vi "RoomJasonTest.vi"() -> (0 "error out":errorcluster, 2 "Pass":bool)   [LabVIEW 2015]
uses:
  Flags/ColorEnum.ctl
  NurseStation/TypeDef/SelectedRoom.ctl
  Flags/ColorFlags.ctl
  Room/Room.lvclass/Room.ctl
  Room/Write Beacon Id.vi
  Room/Write BedVacant.vi
  Room/Write InRoomPersonnel.vi
  Room/Write RoomRequests.vi
  Room/Read Beacon Id.vi
  Room/Read BedVacant.vi
  Room/Read InRoomPersonnel.vi
  Room/Read Room Number.vi
  Room/Read RoomRequests.vi
  Room/Read Flags.lvclass.vi
  Flags/Flags.lvclass
  Room/Room.lvclass
panel:
  out "String":string
  in  "RoomRequests":string[](array[string])=["Cleanning"]
  in  "InRoomPersonnel":string[](array[string])=["Dr Y"]
  in  "BedVacant":bool
  in  "Beacon Id":string="test"
  out "After Json":T1={"Room Number"=0, "RoomNumFlags"={"Flag State"=[1, 3, 5, 7]}, "BedVacant"=FALSE, "InRoomPersonnel"=[], "RoomRequests"=[]}
  out "Before Json":T1={"Room Number"=0, "RoomNumFlags"={"Flag State"=[1, 3, 5, 7]}, "BedVacant"=FALSE, "InRoomPersonnel"=[], "RoomRequests"=[]}
  in  "Color":T3[](array[typedef])=[enum."Red", enum."Blue", enum."Green", enum."Yellow"]
  in  "State":bool[](array[boolean])=[FALSE, FALSE, FALSE, TRUE]
  in  "Room Number":u8=1
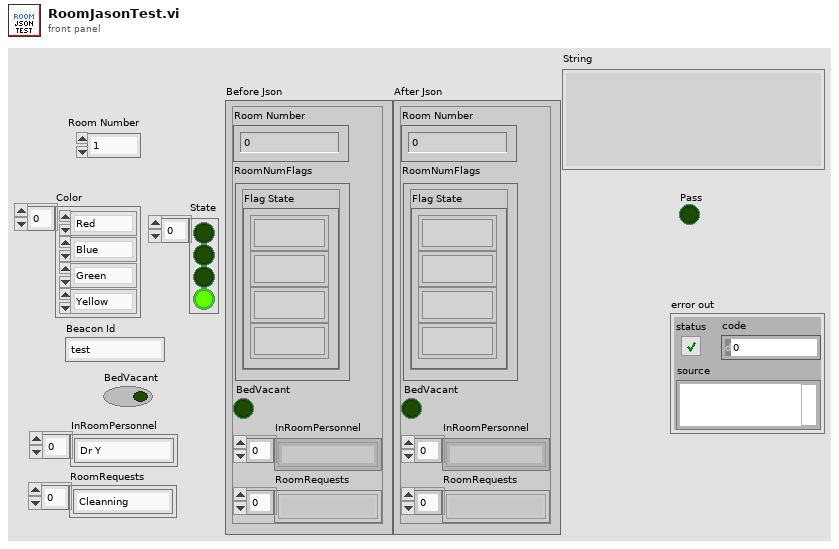
[diagram p1: front panel]
types:
  T1 = typedef "SelectedRoom.ctl" = cluster{"Room Number":u8, "RoomNumFlags":T2, "BedVacant":bool, "InRoomPersonnel":string[], "RoomRequests":string[]}
  T2 = typedef "Flags.lvclass/ColorFlags.ctl" = cluster{"Flag State":u8[]}
  T3 = typedef "Flags.lvclass/ColorEnum.ctl" = enum8{"Red", "Blue", "Green", "Yellow"}
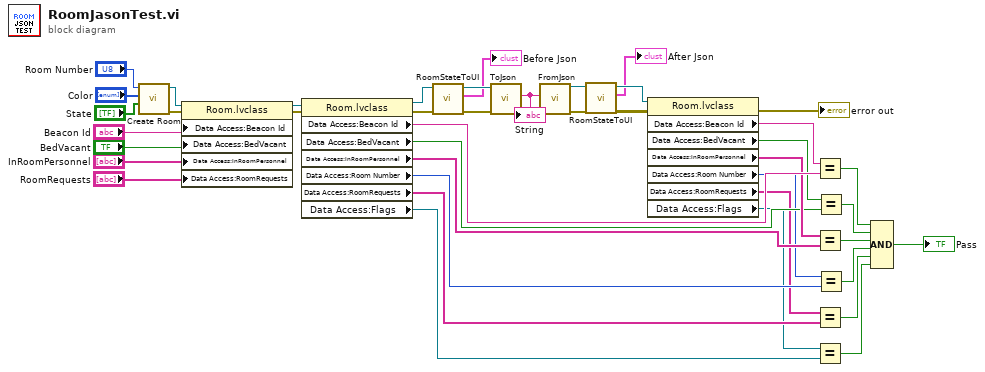
[diagram p0: block diagram]
diagram:
  n1 = call "Create Room.vi"("State"="State", "Color"="Color", "Room Number"="Room Number") -> ("error out"=w7:errorcluster, "Room Ref"=w8:refnum<class "Room.lvclass">)  [unwired: 7 in]
  n2 = property class="Room.lvclass"(reference=w8, error in=w7, "Data Access:Beacon Id"="Beacon Id", "Data Access:BedVacant"="BedVacant", "Data Access:InRoomPersonnel"="InRoomPersonnel", "Data Access:RoomRequests"="RoomRequests") -> (reference out=w6:refnum<class "Room.lvclass">, error out=w5:errorcluster)
  n3 = property class="Room.lvclass"(reference=w6, error in=w5) -> (reference out=w18:refnum<class "Room.lvclass">, error out=w17:errorcluster, "Data Access:Beacon Id"=w42:string, "Data Access:BedVacant"=w36:bool, "Data Access:InRoomPersonnel"=w35:string[], "Data Access:Room Number"=w27:i32, "Data Access:RoomRequests"=w25:string[], "Data Access:Flags"=w21:refnum<class "Flags.lvclass">)
  n4 = call "RoomStateToUI.vi"("error in"=w17, "Room In"=w18) -> ("error out"=w16:errorcluster, "Selected Room"=→"Before Json":T1, "Room Out"=w15:refnum<class "Room.lvclass">)  [unwired: 7 in]
  n5 = call "ToJson.vi"("error in (no error)"=w16, "Room in"=w15) -> ("error out"=w29:errorcluster, "String"=w19:string)  [unwired: 7 in, 1 out]
  "String" <- w19
  n6 = call "FromJson.vi"("error in (no error)"=w29, "String"=w19) -> ("error out"=w14:errorcluster, "Room out"=w11:refnum<class "Room.lvclass">)  [unwired: 8 in]
  n7 = call "RoomStateToUI.vi"("error in"=w14, "Room In"=w11) -> ("error out"=w13:errorcluster, "Selected Room"=→"After Json":T1, "Room Out"=w12:refnum<class "Room.lvclass">)  [unwired: 7 in]
  n8 = property class="Room.lvclass"(reference=w12, error in=w13) -> (error out=→"error out":errorcluster, "Data Access:Beacon Id"=w43:string, "Data Access:BedVacant"=w41:bool, "Data Access:InRoomPersonnel"=w37:string[], "Data Access:Room Number"=w28:i32, "Data Access:RoomRequests"=w26:string[], "Data Access:Flags"=w20:refnum<class "Flags.lvclass">)  [unwired: 1 out]
  n9 = Equal?(x=w43, y=w42) -> (x = y?=w40:bool)
  n10 = Equal?(x=w37, y=w35) -> (x = y?=w33:bool)
  n11 = Equal?(x=w26, y=w25) -> (x = y?=w23:bool)
  n12 = Equal?(x=w20, y=w21) -> (x = y?=w22:bool)
  n13 = Equal?(x=w41, y=w36) -> (x = y?=w34:bool)
  n14 = Equal?(x=w28, y=w27) -> (x = y?=w24:bool)
  n15 = Compound Arithmetic op=AND(w40, w34, w33, w24, w23, w22) -> (→"Pass":bool)
